vi "LabVIEW_Version to LV_VERS and LV_BIT.vi"(11 "Package_LabVIEW_Version":string) -> (2 "LV_BIT":u32(ring)=64 items=["32"=32, "64"=64], 3 "LV_VER":u32)   [LabVIEW 2019, in "PostBuildSupport.lvclass"]
uses:
  PostBuildSupport/PostBuildSupport.lvclass
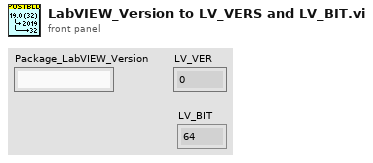
[diagram p1: front panel]
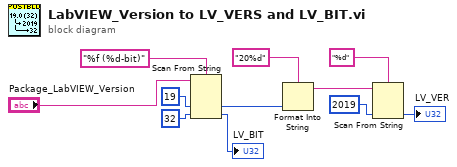
[diagram p0: block diagram]
diagram:
  n1 = Scan From String(format string="%f (%d-bit)", input string="Package_LabVIEW_Version", default 1=u32 19 ("default value 2"), default 2=u32 32 ("default value 2")) -> (output 1=w6:u32, output 2=→"LV_BIT":u32)  [unwired: 2 in, 3 out]
  n2 = Format Into String(format string="20%d", w6) -> (resulting string=w8:string)  [unwired: 2 in, 1 out]
  n3 = Scan From String(format string="%d", input string=w8, default 1=u32 2019 ("default value 2")) -> (output 1=→"LV_VER":u32)  [unwired: 2 in, 3 out]
